vi "Set Double Float.vi"(10 "Value":dbl, 11 "Abs_Double Float.lvclass":refnum<class "Abs_Double Float.lvclass">) -> (3 "Node":refnum<class "bt_Node.lvclass">)   [LabVIEW 2021, in "BT AbsType.lvlib"]
uses:
  BT AbsType.lvlib
  Source/Support/Nodes/abs_Node/bt_Node.lvclass
  <vilib>/TSA/Abstract Data Classes/Abs_Types/Double Float/Abs_Double Float.lvclass
  C:/Program Files (x86)/National Instruments/LabVIEW 2021/vi.lib/TSA/Abstract Data Classes/Abs_Types/Type/Abs_Type.lvclass
  Set Double Float/Set Double Float.lvclass
  C:/Users/Tim/Documents/GitHub/LV_Behaviour_Tree/BT Abstract Type/abs_Type Leaf/abs_Type Leaf.lvclass
  C:/Users/Tim/Documents/GitHub/LV_Behaviour_Tree/Source/Support/Nodes/abs_Node/bt_Node.lvclass
  abs_Type Leaf/abs_Type Leaf.lvclass/abs_Type Leaf.ctl
  Set Double Float/Set Double Float.lvclass/Set Double Float.ctl
  abs_Type Leaf/Properties/Write Value Class.vi
  Set Double Float/Properties/Write Value.vi
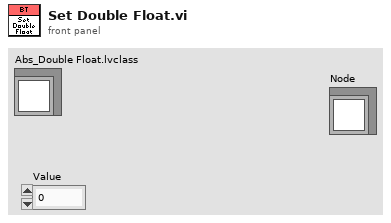
[diagram p1: front panel]
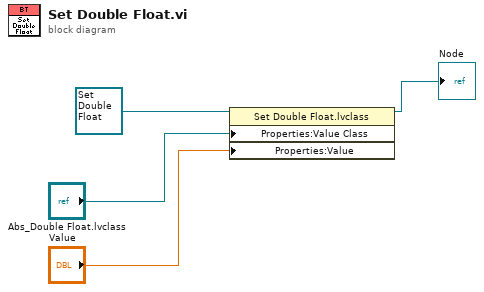
[diagram p0: block diagram]
diagram:
  n1 = property class="Set Double Float.lvclass"(reference=refnum<class "Set Double Float.lvclass"> refnum ("BT.lvlib:Set Double Float.lvclass"), "Properties:Value Class"="Abs_Double Float.lvclass", "Properties:Value"="Value") -> (reference out=→"Node":refnum<class "Set Double Float.lvclass">)  [unwired: 1 in, 1 out]
